vi "Disabled.vi"(7 "Robot Mode":T2, 10 "Match Info":T1={"Autonomous Elapsed Seconds"=0.0, "TeleOp Elapsed Seconds"=0.0, "Disabled Elapsed Seconds"=0.0, "Visited Autonomous"=FALSE, "Visited TeleOp"=FALSE, "Visited Disabled"=FALSE, "Autonomous Settings"={"Autonomous Style"=enum."Independent", "VI Refnum"=refnum}}, 11 "Call Context":T3) -> ()   [LabVIEW 2017]
doc: "This VI is called each time a disabled packet is received from the DS. It is often used to prepare for the next robot mode, to calibrate sensors, etc."
uses:
  <vilib>/Rock Robotics/WPI/DriverStation/WPI_DriverStationDerivedRobotMode.ctl
  <vilib>/Rock Robotics/WPI/DriverStation/WPI_DriverStationRobotMode2.ctl
  <vilib>/Rock Robotics/WPI/DriverStation/WPI_DriverStationMatch Info.ctl
  <vilib>/Rock Robotics/Network Tables/NT Write String Array.vi
  <vilib>/Rock Robotics/Network Tables/NT Write Numeric Array.vi
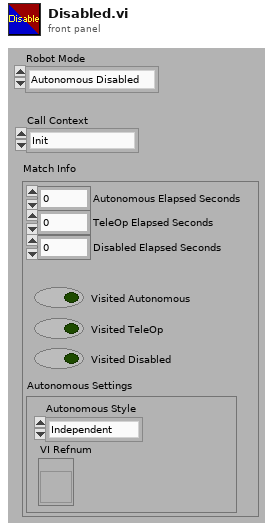
[diagram p1: front panel]
types:
  T1 = typedef "WPI_DriverStationMatch Info.ctl" = cluster{"Autonomous Elapsed Seconds":dbl, "TeleOp Elapsed Seconds":dbl, "Disabled Elapsed Seconds":dbl, "Visited Autonomous":bool, "Visited TeleOp":bool, "Visited Disabled":bool, "Autonomous Settings":cluster{"Autonomous Style":enum16{"Iterative", "Independent"}, "VI Refnum":refnum<vi>}}
  T2 = typedef "WPI_DriverStationRobotMode2.ctl" = enum16{"Autonomous Disabled", "Autonomous Enabled", "Teleop Disabled", "Teleop Enabled", "Disconnected", "Finish", "Test Disabled", "Test Enabled", "Emergency Stopped"}
  T3 = typedef "WPI_DriverStationDerivedRobotMode.ctl" = enum16{"Init", "Execute", "Stop"}
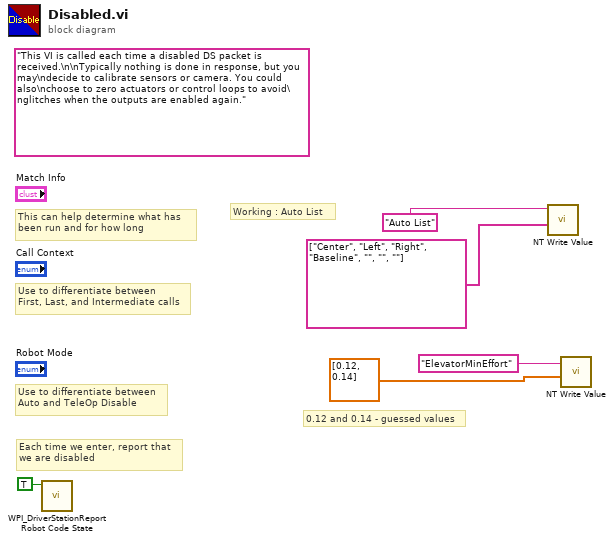
[diagram p0: block diagram]
diagram:
  (unwired) "This VI is called each time a disabled DS packet is received.\n\nTypically nothing is done in response, but you may\ndecide to calibrate sensors or camera. You could also\nchoose to zero actuators or control loops to avoid\nglitches when the outputs are enabled again."
  # "0.12 and 0.14 - guessed values"
  # "Working : Auto List"
  # "Each time we enter, report that\nwe are disabled"
  # "Use to differentiate between\nFirst, Last, and Intermediate calls"
  # "This can help determine what has\nbeen run and for how long"
  # "Use to differentiate between\nAuto and TeleOp Disable"
  n1 = call <vilib>:"WPI_DriverStationReport Robot Code State.vi"("Disabled"=TRUE ("Autonomous")) -> ()  [unwired: 10 in, 1 out]
  n2 = call-poly <vilib>:"NT Write Value.vi"("String Array"=string[] ["Center", "Left", "Right", "Baseline", "", "", ""], "Name"="Auto List") -> ()  [unwired: 9 in, 1 out]
  n3 = call-poly <vilib>:"NT Write Value.vi"("Numeric Array"=dbl[] [0.12, 0.14] ("Array - Numeric"), "Name"="ElevatorMinEffort") -> ()  [unwired: 9 in, 1 out]
